vi "DDS_Clock.vi"() -> ()   [LabVIEW 2016] (continued)
{"STEP"=0, "time[ms]"=0.05, "time tolerance[us]"=0.01, "CH0"=TRUE, "rel. amplitude CH0"=1.0, "phase [°] CH0"=0.0, "f0 [Hz] CH0"=304600000.0, "f1 [Hz] CH0"=304400000.0, "CH1"=FALSE, "rel. amplitude CH1"=1.0, "phase [°] CH1"=0.0, "f0 [Hz] CH1"=310000000.0, "f1 [Hz] CH1"=310000000.0}, {"STEP"=0, "time[ms]"=0.05, "time tolerance[us]"=0.01, "CH0"=TRUE, "rel. amplitude CH0"=1.0, "phase [°] CH0"=0.0, "f0 [Hz] CH0"=304400000.0, "f1 [Hz] CH0"=304200000.0, "CH1"=FALSE, "rel. amplitude CH1"=1.0, "phase [°] CH1"=0.0, "f0 [Hz] CH1"=310000000.0, "f1 [Hz] CH1"=310000000.0}, {"STEP"=0, "time[ms]"=0.05, "time tolerance[us]"=0.01, "CH0"=TRUE, "rel. amplitude CH0"=1.0, "phase [°] CH0"=0.0, "f0 [Hz] CH0"=304200000.0, "f1 [Hz] CH0"=304000000.0, "CH1"=FALSE, "rel. amplitude CH1"=1.0, "phase [°] CH1"=0.0, "f0 [Hz] CH1"=310000000.0, "f1 [Hz] CH1"=310000000.0}, {"STEP"=0, "time[ms]"=0.05, "time tolerance[us]"=0.01, "CH0"=TRUE, "rel. amplitude CH0"=1.0, "phase [°] CH0"=0.0, "f0 [Hz] CH0"=304000000.0, "f1 [Hz] CH0"=303800000.0, "CH1"=FALSE, "rel. amplitude CH1"=1.0, "phase [°] CH1"=0.0, "f0 [Hz] CH1"=310000000.0, "f1 [Hz] CH1"=310000000.0}, {"STEP"=0, "time[ms]"=0.05, "time tolerance[us]"=0.01, "CH0"=TRUE, "rel. amplitude CH0"=1.0, "phase [°] CH0"=0.0, "f0 [Hz] CH0"=303800000.0, "f1 [Hz] CH0"=303600000.0, "CH1"=FALSE, "rel. amplitude CH1"=1.0, "phase [°] CH1"=0.0, "f0 [Hz] CH1"=310000000.0, "f1 [Hz] CH1"=310000000.0}, {"STEP"=0, "time[ms]"=0.05, "time tolerance[us]"=0.01, "CH0"=TRUE, "rel. amplitude CH0"=1.0, "phase [°] CH0"=0.0, "f0 [Hz] CH0"=303600000.0, "f1 [Hz] CH0"=303399999.99999994, "CH1"=FALSE, "rel. amplitude CH1"=1.0, "phase [°] CH1"=0.0, "f0 [Hz] CH1"=310000000.0, "f1 [Hz] CH1"=310000000.0}, {"STEP"=0, "time[ms]"=0.05, "time tolerance[us]"=0.01, "CH0"=TRUE, "rel. amplitude CH0"=1.0, "phase [°] CH0"=0.0, "f0 [Hz] CH0"=303399999.99999994, "f1 [Hz] CH0"=303200000.0, "CH1"=FALSE, "rel. amplitude CH1"=1.0, "phase [°] CH1"=0.0, "f0 [Hz] CH1"=310000000.0, "f1 [Hz] CH1"=310000000.0}, {"STEP"=0, "time[ms]"=0.05, "time tolerance[us]"=0.01, "CH0"=TRUE, "rel. amplitude CH0"=1.0, "phase [°] CH0"=0.0, "f0 [Hz] CH0"=303200000.0, "f1 [Hz] CH0"=303000000.0, "CH1"=FALSE, "rel. amplitude CH1"=1.0, "phase [°] CH1"=0.0, "f0 [Hz] CH1"=310000000.0, "f1 [Hz] CH1"=310000000.0}, {"STEP"=0, "time[ms]"=0.05, "time tolerance[us]"=0.01, "CH0"=TRUE, "rel. amplitude CH0"=1.0, "phase [°] CH0"=0.0, "f0 [Hz] CH0"=303000000.0, "f1 [Hz] CH0"=302800000.0, "CH1"=FALSE, "rel. amplitude CH1"=1.0, "phase [°] CH1"=0.0, "f0 [Hz] CH1"=310000000.0, "f1 [Hz] CH1"=310000000.0}, {"STEP"=0, "time[ms]"=0.05, "time tolerance[us]"=0.01, "CH0"=TRUE, "rel. amplitude CH0"=1.0, "phase [°] CH0"=0.0, "f0 [Hz] CH0"=302800000.0, "f1 [Hz] CH0"=302600000.0, "CH1"=FALSE, "rel. amplitude CH1"=1.0, "phase [°] CH1"=0.0, "f0 [Hz] CH1"=310000000.0, "f1 [Hz] CH1"=310000000.0}, {"STEP"=0, "time[ms]"=0.05, "time tolerance[us]"=0.01, "CH0"=TRUE, "rel. amplitude CH0"=1.0, "phase [°] CH0"=0.0, "f0 [Hz] CH0"=302600000.0, "f1 [Hz] CH0"=302399999.99999994, "CH1"=FALSE, "rel. amplitude CH1"=1.0, "phase [°] CH1"=0.0, "f0 [Hz] CH1"=310000000.0, "f1 [Hz] CH1"=310000000.0}, {"STEP"=0, "time[ms]"=0.05, "time tolerance[us]"=0.01, "CH0"=TRUE, "rel. amplitude CH0"=1.0, "phase [°] CH0"=0.0, "f0 [Hz] CH0"=302399999.99999994, "f1 [Hz] CH0"=302200000.0, "CH1"=FALSE, "rel. amplitude CH1"=1.0, "phase [°] CH1"=0.0, "f0 [Hz] CH1"=310000000.0, "f1 [Hz] CH1"=310000000.0}, {"STEP"=0, "time[ms]"=0.05, "time tolerance[us]"=0.01, "CH0"=TRUE, "rel. amplitude CH0"=1.0, "phase [°] CH0"=0.0, "f0 [Hz] CH0"=302200000.0, "f1 [Hz] CH0"=302000000.0, "CH1"=FALSE, "rel. amplitude CH1"=1.0, "phase [°] CH1"=0.0, "f0 [Hz] CH1"=310000000.0, "f1 [Hz] CH1"=310000000.0}, {"STEP"=0, "time[ms]"=0.05, "time tolerance[us]"=0.01, "CH0"=TRUE, "rel. amplitude CH0"=1.0, "phase [°] CH0"=0.0, "f0 [Hz] CH0"=302000000.0, "f1 [Hz] CH0"=301800000.0, "CH1"=FALSE, "rel. amplitude CH1"=1.0, "phase [°] CH1"=0.0, "f0 [Hz] CH1"=310000000.0, "f1 [Hz] CH1"=310000000.0}, {"STEP"=0, "time[ms]"=0.05, "time tolerance[us]"=0.01, "CH0"=TRUE, "rel. amplitude CH0"=1.0, "phase [°] CH0"=0.0, "f0 [Hz] CH0"=301800000.0, "f1 [Hz] CH0"=301600000.0, "CH1"=FALSE, "rel. amplitude CH1"=1.0, "phase [°] CH1"=0.0, "f0 [Hz] CH1"=310000000.0, "f1 [Hz] CH1"=310000000.0}, {"STEP"=0, "time[ms]"=0.05, "time tolerance[us]"=0.01, "CH0"=TRUE, "rel. amplitude CH0"=1.0, "phase [°] CH0"=0.0, "f0 [Hz] CH0"=301600000.0, "f1 [Hz] CH0"=301400000.0, "CH1"=FALSE, "rel. amplitude CH1"=1.0, "phase [°] CH1"=0.0, "f0 [Hz] CH1"=310000000.0, "f1 [Hz] CH1"=310000000.0}, {"STEP"=0, "time[ms]"=0.05, "time tolerance[us]"=0.01, "CH0"=TRUE, "rel. amplitude CH0"=1.0, "phase [°] CH0"=0.0, "f0 [Hz] CH0"=301400000.0, "f1 [Hz] CH0"=301200000.0, "CH1"=FALSE, "rel. amplitude CH1"=1.0, "phase [°] CH1"=0.0, "f0 [Hz] CH1"=310000000.0, "f1 [Hz] CH1"=310000000.0}, {"STEP"=0, "time[ms]"=0.05, "time tolerance[us]"=0.01, "CH0"=TRUE, "rel. amplitude CH0"=1.0, "phase [°] CH0"=0.0, "f0 [Hz] CH0"=301200000.0, "f1 [Hz] CH0"=301000000.0, "CH1"=FALSE, "rel. amplitude CH1"=1.0, "phase [°] CH1"=0.0, "f0 [Hz] CH1"=310000000.0, "f1 [Hz] CH1"=310000000.0}, {"STEP"=0, "time[ms]"=0.05, "time tolerance[us]"=0.01, "CH0"=TRUE, "rel. amplitude CH0"=1.0, "phase [°] CH0"=0.0, "f0 [Hz] CH0"=301000000.0, "f1 [Hz] CH0"=300800000.0, "CH1"=FALSE, "rel. amplitude CH1"=1.0, "phase [°] CH1"=0.0, "f0 [Hz] CH1"=310000000.0, "f1 [Hz] CH1"=310000000.0}, {"STEP"=0, "time[ms]"=0.05, "time tolerance[us]"=0.01, "CH0"=TRUE, "rel. amplitude CH0"=1.0, "phase [°] CH0"=0.0, "f0 [Hz] CH0"=300800000.0, "f1 [Hz] CH0"=300600000.0, "CH1"=FALSE, "rel. amplitude CH1"=1.0, "phase [°] CH1"=0.0, "f0 [Hz] CH1"=310000000.0, "f1 [Hz] CH1"=310000000.0}, {"STEP"=0, "time[ms]"=0.05, "time tolerance[us]"=0.01, "CH0"=TRUE, "rel. amplitude CH0"=1.0, "phase [°] CH0"=0.0, "f0 [Hz] CH0"=300600000.0, "f1 [Hz] CH0"=300400000.0, "CH1"=FALSE, "rel. amplitude CH1"=1.0, "phase [°] CH1"=0.0, "f0 [Hz] CH1"=310000000.0, "f1 [Hz] CH1"=310000000.0}, {"STEP"=0, "time[ms]"=0.05, "time tolerance[us]"=0.01, "CH0"=TRUE, "rel. amplitude CH0"=1.0, "phase [°] CH0"=0.0, "f0 [Hz] CH0"=300400000.0, "f1 [Hz] CH0"=300200000.0, "CH1"=FALSE, "rel. amplitude CH1"=1.0, "phase [°] CH1"=0.0, "f0 [Hz] CH1"=310000000.0, "f1 [Hz] CH1"=310000000.0}, {"STEP"=0, "time[ms]"=0.05, "time tolerance[us]"=0.01, "CH0"=TRUE, "rel. amplitude CH0"=1.0, "phase [°] CH0"=0.0, "f0 [Hz] CH0"=300200000.0, "f1 [Hz] CH0"=300000000.0, "CH1"=FALSE, "rel. amplitude CH1"=1.0, "phase [°] CH1"=0.0, "f0 [Hz] CH1"=310000000.0, "f1 [Hz] CH1"=310000000.0}, {"STEP"=0, "time[ms]"=0.05, "time tolerance[us]"=0.01, "CH0"=TRUE, "rel. amplitude CH0"=1.0, "phase [°] CH0"=0.0, "f0 [Hz] CH0"=300000000.0, "f1 [Hz] CH0"=300200000.00000006, "CH1"=FALSE, "rel. amplitude CH1"=1.0, "phase [°] CH1"=0.0, "f0 [Hz] CH1"=310000000.0, "f1 [Hz] CH1"=310000000.0}, {"STEP"=0, "time[ms]"=0.05, "time tolerance[us]"=0.01, "CH0"=TRUE, "rel. amplitude CH0"=1.0, "phase [°] CH0"=0.0, "f0 [Hz] CH0"=300200000.00000006, "f1 [Hz] CH0"=300400000.0, "CH1"=FALSE, "rel. amplitude CH1"=1.0, "phase [°] CH1"=0.0, "f0 [Hz] CH1"=310000000.0, "f1 [Hz] CH1"=310000000.0}, {"STEP"=0, "time[ms]"=0.05, "time tolerance[us]"=0.01, "CH0"=TRUE, "rel. amplitude CH0"=1.0, "phase [°] CH0"=0.0, "f0 [Hz] CH0"=300400000.0, "f1 [Hz] CH0"=300600000.0, "CH1"=FALSE, "rel. amplitude CH1"=1.0, "phase [°] CH1"=0.0, "f0 [Hz] CH1"=310000000.0, "f1 [Hz] CH1"=310000000.0}, {"STEP"=0, "time[ms]"=0.05, "time tolerance[us]"=0.01, "CH0"=TRUE, "rel. amplitude CH0"=1.0, "phase [°] CH0"=0.0, "f0 [Hz] CH0"=300600000.0, "f1 [Hz] CH0"=300800000.0, "CH1"=FALSE, "rel. amplitude CH1"=1.0, "phase [°] CH1"=0.0, "f0 [Hz] CH1"=310000000.0, "f1 [Hz] CH1"=310000000.0}, {"STEP"=0, "time[ms]"=0.05, "time tolerance[us]"=0.01, "CH0"=TRUE, "rel. amplitude CH0"=1.0, "phase [°] CH0"=0.0, "f0 [Hz] CH0"=300800000.0, "f1 [Hz] CH0"=301000000.0, "CH1"=FALSE, "rel. amplitude CH1"=1.0, "phase [°] CH1"=0.0, "f0 [Hz] CH1"=310000000.0, "f1 [Hz] CH1"=310000000.0}, {"STEP"=0, "time[ms]"=0.05, "time tolerance[us]"=0.01, "CH0"=TRUE, "rel. amplitude CH0"=1.0, "phase [°] CH0"=0.0, "f0 [Hz] CH0"=301000000.0, "f1 [Hz] CH0"=301200000.0, "CH1"=FALSE, "rel. amplitude CH1"=1.0, "phase [°] CH1"=0.0, "f0 [Hz] CH1"=310000000.0, "f1 [Hz] CH1"=310000000.0}, {"STEP"=0, "time[ms]"=0.05, "time tolerance[us]"=0.01, "CH0"=TRUE, "rel. amplitude CH0"=1.0, "phase [°] CH0"=0.0, "f0 [Hz] CH0"=301200000.0, "f1 [Hz] CH0"=301400000.0, "CH1"=FALSE, "rel. amplitude CH1"=1.0, "phase [°] CH1"=0.0, "f0 [Hz] CH1"=310000000.0, "f1 [Hz] CH1"=310000000.0}, {"STEP"=0, "time[ms]"=0.05, "time tolerance[us]"=0.01, "CH0"=TRUE, "rel. amplitude CH0"=1.0, "phase [°] CH0"=0.0, "f0 [Hz] CH0"=301400000.0, "f1 [Hz] CH0"=301600000.00000006, "CH1"=FALSE, "rel. amplitude CH1"=1.0, "phase [°] CH1"=0.0, "f0 [Hz] CH1"=310000000.0, "f1 [Hz] CH1"=310000000.0}, {"STEP"=0, "time[ms]"=0.05, "time tolerance[us]"=0.01, "CH0"=TRUE, "rel. amplitude CH0"=1.0, "phase [°] CH0"=0.0, "f0 [Hz] CH0"=301600000.00000006, "f1 [Hz] CH0"=301800000.00000006, "CH1"=FALSE, "rel. amplitude CH1"=1.0, "phase [°] CH1"=0.0, "f0 [Hz] CH1"=310000000.0, "f1 [Hz] CH1"=310000000.0}, {"STEP"=0, "time[ms]"=0.05, "time tolerance[us]"=0.01, "CH0"=TRUE, "rel. amplitude CH0"=1.0, "phase [°] CH0"=0.0, "f0 [Hz] CH0"=301800000.00000006, "f1 [Hz] CH0"=302000000.0, "CH1"=FALSE, "rel. amplitude CH1"=1.0, "phase [°] CH1"=0.0, "f0 [Hz] CH1"=310000000.0, "f1 [Hz] CH1"=310000000.0}, {"STEP"=0, "time[ms]"=0.05, "time tolerance[us]"=0.01, "CH0"=TRUE, "rel. amplitude CH0"=1.0, "phase [°] CH0"=0.0, "f0 [Hz] CH0"=302000000.0, "f1 [Hz] CH0"=302200000.0, "CH1"=FALSE, "rel. amplitude CH1"=1.0, "phase [°] CH1"=0.0, "f0 [Hz] CH1"=310000000.0, "f1 [Hz] CH1"=310000000.0}, {"STEP"=0, "time[ms]"=0.05, "time tolerance[us]"=0.01, "CH0"=TRUE, "rel. amplitude CH0"=1.0, "phase [°] CH0"=0.0, "f0 [Hz] CH0"=302200000.0, "f1 [Hz] CH0"=302400000.0, "CH1"=FALSE, "rel. amplitude CH1"=1.0, "phase [°] CH1"=0.0, "f0 [Hz] CH1"=310000000.0, "f1 [Hz] CH1"=310000000.0}, {"STEP"=0, "time[ms]"=0.05, "time tolerance[us]"=0.01, "CH0"=TRUE, "rel. amplitude CH0"=1.0, "phase [°] CH0"=0.0, "f0 [Hz] CH0"=302400000.0, "f1 [Hz] CH0"=302600000.0, "CH1"=FALSE, "rel. amplitude CH1"=1.0, "phase [°] CH1"=0.0, "f0 [Hz] CH1"=310000000.0, "f1 [Hz] CH1"=310000000.0}, {"STEP"=0, "time[ms]"=0.05, "time tolerance[us]"=0.01, "CH0"=TRUE, "rel. amplitude CH0"=1.0, "phase [°] CH0"=0.0, "f0 [Hz] CH0"=302600000.0, "f1 [Hz] CH0"=302800000.0, "CH1"=FALSE, "rel. amplitude CH1"=1.0, "phase [°] CH1"=0.0, "f0 [Hz] CH1"=310000000.0, "f1 [Hz] CH1"=310000000.0}, {"STEP"=0, "time[ms]"=0.05, "time tolerance[us]"=0.01, "CH0"=TRUE, "rel. amplitude CH0"=1.0, "phase [°] CH0"=0.0, "f0 [Hz] CH0"=302800000.0, "f1 [Hz] CH0"=303000000.0, "CH1"=FALSE, "rel. amplitude CH1"=1.0, "phase [°] CH1"=0.0, "f0 [Hz] CH1"=310000000.0, "f1 [Hz] CH1"=310000000.0}, {"STEP"=0, "time[ms]"=0.05, "time tolerance[us]"=0.01, "CH0"=TRUE, "rel. amplitude CH0"=1.0, "phase [°] CH0"=0.0, "f0 [Hz] CH0"=303000000.0, "f1 [Hz] CH0"=303200000.00000006, "CH1"=FALSE, "rel. amplitude CH1"=1.0, "phase [°] CH1"=0.0, "f0 [Hz] CH1"=310000000.0, "f1 [Hz] CH1"=310000000.0}, {"STEP"=0, "time[ms]"=0.05, "time tolerance[us]"=0.01, "CH0"=TRUE, "rel. amplitude CH0"=1.0, "phase [°] CH0"=0.0, "f0 [Hz] CH0"=303200000.00000006, "f1 [Hz] CH0"=303400000.0, "CH1"=FALSE, "rel. amplitude CH1"=1.0, "phase [°] CH1"=0.0, "f0 [Hz] CH1"=310000000.0, "f1 [Hz] CH1"=310000000.0}, {"STEP"=0, "time[ms]"=0.05, "time tolerance[us]"=0.01, "CH0"=TRUE, "rel. amplitude CH0"=1.0, "phase [°] CH0"=0.0, "f0 [Hz] CH0"=303400000.0, "f1 [Hz] CH0"=303600000.0, "CH1"=FALSE, "rel. amplitude CH1"=1.0, "phase [°] CH1"=0.0, "f0 [Hz] CH1"=310000000.0, "f1 [Hz] CH1"=310000000.0}, {"STEP"=0, "time[ms]"=0.05, "time tolerance[us]"=0.01, "CH0"=TRUE, "rel. amplitude CH0"=1.0, "phase [°] CH0"=0.0, "f0 [Hz] CH0"=303600000.0, "f1 [Hz] CH0"=303800000.0, "CH1"=FALSE, "rel. amplitude CH1"=1.0, "phase [°] CH1"=0.0, "f0 [Hz] CH1"=310000000.0, "f1 [Hz] CH1"=310000000.0}, {"STEP"=0, "time[ms]"=0.05, "time tolerance[us]"=0.01, "CH0"=TRUE, "rel. amplitude CH0"=1.0, "phase [°] CH0"=0.0, "f0 [Hz] CH0"=303800000.0, "f1 [Hz] CH0"=304000000.0, "CH1"=FALSE, "rel. amplitude CH1"=1.0, "phase [°] CH1"=0.0, "f0 [Hz] CH1"=310000000.0, "f1 [Hz] CH1"=310000000.0}, {"STEP"=0, "time[ms]"=0.05, "time tolerance[us]"=0.01, "CH0"=TRUE, "rel. amplitude CH0"=1.0, "phase [°] CH0"=0.0, "f0 [Hz] CH0"=304000000.0, "f1 [Hz] CH0"=304200000.0, "CH1"=FALSE, "rel. amplitude CH1"=1.0, "phase [°] CH1"=0.0, "f0 [Hz] CH1"=310000000.0, "f1 [Hz] CH1"=310000000.0}, {"STEP"=0, "time[ms]"=0.05, "time tolerance[us]"=0.01, "CH0"=TRUE, "rel. amplitude CH0"=1.0, "phase [°] CH0"=0.0, "f0 [Hz] CH0"=304200000.0, "f1 [Hz] CH0"=304400000.0, "CH1"=FALSE, "rel. amplitude CH1"=1.0, "phase [°] CH1"=0.0, "f0 [Hz] CH1"=310000000.0, "f1 [Hz] CH1"=310000000.0}, {"STEP"=0, "time[ms]"=0.05, "time tolerance[us]"=0.01, "CH0"=TRUE, "rel. amplitude CH0"=1.0, "phase [°] CH0"=0.0, "f0 [Hz] CH0"=304400000.0, "f1 [Hz] CH0"=304600000.00000006, "CH1"=FALSE, "rel. amplitude CH1"=1.0, "phase [°] CH1"=0.0, "f0 [Hz] CH1"=310000000.0, "f1 [Hz] CH1"=310000000.0}, {"STEP"=0, "time[ms]"=0.05, "time tolerance[us]"=0.01, "CH0"=TRUE, "rel. amplitude CH0"=1.0, "phase [°] CH0"=0.0, "f0 [Hz] CH0"=304600000.00000006, "f1 [Hz] CH0"=304800000.0, "CH1"=FALSE, "rel. amplitude CH1"=1.0, "phase [°] CH1"=0.0, "f0 [Hz] CH1"=310000000.0, "f1 [Hz] CH1"=310000000.0}, {"STEP"=0, "time[ms]"=0.05, "time tolerance[us]"=0.01, "CH0"=TRUE, "rel. amplitude CH0"=1.0, "phase [°] CH0"=0.0, "f0 [Hz] CH0"=304800000.0, "f1 [Hz] CH0"=305000000.0, "CH1"=FALSE, "rel. amplitude CH1"=1.0, "phase [°] CH1"=0.0, "f0 [Hz] CH1"=310000000.0, "f1 [Hz] CH1"=310000000.0}, {"STEP"=0, "time[ms]"=0.05, "time tolerance[us]"=0.01, "CH0"=TRUE, "rel. amplitude CH0"=1.0, "phase [°] CH0"=0.0, "f0 [Hz] CH0"=305000000.0, "f1 [Hz] CH0"=305200000.00000006, "CH1"=FALSE, "rel. amplitude CH1"=1.0, "phase [°] CH1"=0.0, "f0 [Hz] CH1"=310000000.0, "f1 [Hz] CH1"=310000000.0}, {"STEP"=0, "time[ms]"=0.05, "time tolerance[us]"=0.01, "CH0"=TRUE, "rel. amplitude CH0"=1.0, "phase [°] CH0"=0.0, "f0 [Hz] CH0"=305200000.00000006, "f1 [Hz] CH0"=305400000.0, "CH1"=FALSE, "rel. amplitude CH1"=1.0, "phase [°] CH1"=0.0, "f0 [Hz] CH1"=310000000.0, "f1 [Hz] CH1"=310000000.0}, {"STEP"=0, "time[ms]"=0.05, "time tolerance[us]"=0.01, "CH0"=TRUE, "rel. amplitude CH0"=1.0, "phase [°] CH0"=0.0, "f0 [Hz] CH0"=305400000.0, "f1 [Hz] CH0"=305600000.0, "CH1"=FALSE, "rel. amplitude CH1"=1.0, "phase [°] CH1"=0.0, "f0 [Hz] CH1"=310000000.0, "f1 [Hz] CH1"=310000000.0}, {"STEP"=0, "time[ms]"=0.05, "time tolerance[us]"=0.01, "CH0"=TRUE, "rel. amplitude CH0"=1.0, "phase [°] CH0"=0.0, "f0 [Hz] CH0"=305600000.0, "f1 [Hz] CH0"=305800000.0, "CH1"=FALSE, "rel. amplitude CH1"=1.0, "phase [°] CH1"=0.0, "f0 [Hz] CH1"=310000000.0, "f1 [Hz] CH1"=310000000.0}, {"STEP"=0, "time[ms]"=0.05, "time tolerance[us]"=0.01, "CH0"=TRUE, "rel. amplitude CH0"=1.0, "phase [°] CH0"=0.0, "f0 [Hz] CH0"=305800000.0, "f1 [Hz] CH0"=306000000.0, "CH1"=FALSE, "rel. amplitude CH1"=1.0, "phase [°] CH1"=0.0, "f0 [Hz] CH1"=310000000.0, "f1 [Hz] CH1"=310000000.0}, {"STEP"=0, "time[ms]"=0.05, "time tolerance[us]"=0.01, "CH0"=TRUE, "rel. amplitude CH0"=1.0, "phase [°] CH0"=0.0, "f0 [Hz] CH0"=306000000.0, "f1 [Hz] CH0"=306200000.0, "CH1"=FALSE, "rel. amplitude CH1"=1.0, "phase [°] CH1"=0.0, "f0 [Hz] CH1"=310000000.0, "f1 [Hz] CH1"=310000000.0}, {"STEP"=0, "time[ms]"=0.05, "time tolerance[us]"=0.01, "CH0"=TRUE, "rel. amplitude CH0"=1.0, "phase [°] CH0"=0.0, "f0 [Hz] CH0"=306200000.0, "f1 [Hz] CH0"=306400000.0, "CH1"=FALSE, "rel. amplitude CH1"=1.0, "phase [°] CH1"=0.0, "f0 [Hz] CH1"=310000000.0, "f1 [Hz] CH1"=310000000.0}, {"STEP"=0, "time[ms]"=0.05, "time tolerance[us]"=0.01, "CH0"=TRUE, "rel. amplitude CH0"=1.0, "phase [°] CH0"=0.0, "f0 [Hz] CH0"=306400000.0, "f1 [Hz] CH0"=306600000.00000006, "CH1"=FALSE, "rel. amplitude CH1"=1.0, "phase [°] CH1"=0.0, "f0 [Hz] CH1"=310000000.0, "f1 [Hz] CH1"=310000000.0}, {"STEP"=0, "time[ms]"=0.05, "time tolerance[us]"=0.01, "CH0"=TRUE, "rel. amplitude CH0"=1.0, "phase [°] CH0"=0.0, "f0 [Hz] CH0"=306600000.00000006, "f1 [Hz] CH0"=306800000.00000006, "CH1"=FALSE, "rel. amplitude CH1"=1.0, "phase [°] CH1"=0.0, "f0 [Hz] CH1"=310000000.0, "f1 [Hz] CH1"=310000000.0}, {"STEP"=0, "time[ms]"=0.05, "time tolerance[us]"=0.01, "CH0"=TRUE, "rel. amplitude CH0"=1.0, "phase [°] CH0"=0.0, "f0 [Hz] CH0"=306800000.00000006, "f1 [Hz] CH0"=307000000.0, "CH1"=FALSE, "rel. amplitude CH1"=1.0, "phase [°] CH1"=0.0, "f0 [Hz] CH1"=310000000.0, "f1 [Hz] CH1"=310000000.0}, {"STEP"=0, "time[ms]"=0.05, "time tolerance[us]"=0.01, "CH0"=TRUE, "rel. amplitude CH0"=1.0, "phase [°] CH0"=0.0, "f0 [Hz] CH0"=307000000.0, "f1 [Hz] CH0"=307200000.0, "CH1"=FALSE, "rel. amplitude CH1"=1.0, "phase [°] CH1"=0.0, "f0 [Hz] CH1"=310000000.0, "f1 [Hz] CH1"=310000000.0}, {"STEP"=0, "time[ms]"=0.05, "time tolerance[us]"=0.01, "CH0"=TRUE, "rel. amplitude CH0"=1.0, "phase [°] CH0"=0.0, "f0 [Hz] CH0"=307200000.0, "f1 [Hz] CH0"=307400000.0, "CH1"=FALSE, "rel. amplitude CH1"=1.0, "phase [°] CH1"=0.0, "f0 [Hz] CH1"=310000000.0, "f1 [Hz] CH1"=310000000.0}, {"STEP"=0, "time[ms]"=0.05, "time tolerance[us]"=0.01, "CH0"=TRUE, "rel. amplitude CH0"=1.0, "phase [°] CH0"=0.0, "f0 [Hz] CH0"=307400000.0, "f1 [Hz] CH0"=307600000.0, "CH1"=FALSE, "rel. amplitude CH1"=1.0, "phase [°] CH1"=0.0, "f0 [Hz] CH1"=310000000.0, "f1 [Hz] CH1"=310000000.0}, {"STEP"=0, "time[ms]"=0.05, "time tolerance[us]"=0.01, "CH0"=TRUE, "rel. amplitude CH0"=1.0, "phase [°] CH0"=0.0, "f0 [Hz] CH0"=307600000.0, "f1 [Hz] CH0"=307800000.0, "CH1"=FALSE, "rel. amplitude CH1"=1.0, "phase [°] CH1"=0.0, "f0 [Hz] CH1"=310000000.0, "f1 [Hz] CH1"=310000000.0}, {"STEP"=0, "time[ms]"=0.05, "time tolerance[us]"=0.01, "CH0"=TRUE, "rel. amplitude CH0"=1.0, "phase [°] CH0"=0.0, "f0 [Hz] CH0"=307800000.0, "f1 [Hz] CH0"=308000000.0, "CH1"=FALSE, "rel. amplitude CH1"=1.0, "phase [°] CH1"=0.0, "f0 [Hz] CH1"=310000000.0, "f1 [Hz] CH1"=310000000.0}, {"STEP"=0, "time[ms]"=0.05, "time tolerance[us]"=0.01, "CH0"=TRUE, "rel. amplitude CH0"=1.0, "phase [°] CH0"=0.0, "f0 [Hz] CH0"=308000000.0, "f1 [Hz] CH0"=308200000.00000006, "CH1"=FALSE, "rel. amplitude CH1"=1.0, "phase [°] CH1"=0.0, "f0 [Hz] CH1"=310000000.0, "f1 [Hz] CH1"=310000000.0}, {"STEP"=0, "time[ms]"=0.05, "time tolerance[us]"=0.01, "CH0"=TRUE, "rel. amplitude CH0"=1.0, "phase [°] CH0"=0.0, "f0 [Hz] CH0"=308200000.00000006, "f1 [Hz] CH0"=308400000.0, "CH1"=FALSE, "rel. amplitude CH1"=1.0, "phase [°] CH1"=0.0, "f0 [Hz] CH1"=310000000.0, "f1 [Hz] CH1"=310000000.0}, {"STEP"=0, "time[ms]"=0.05, "time tolerance[us]"=0.01, "CH0"=TRUE, "rel. amplitude CH0"=1.0, "phase [°] CH0"=0.0, "f0 [Hz] CH0"=308400000.0, "f1 [Hz] CH0"=308600000.0, "CH1"=FALSE, "rel. amplitude CH1"=1.0, "phase [°] CH1"=0.0, "f0 [Hz] CH1"=310000000.0, "f1 [Hz] CH1"=310000000.0}, {"STEP"=0, "time[ms]"=0.05, "time tolerance[us]"=0.01, "CH0"=TRUE, "rel. amplitude CH0"=1.0, "phase [°] CH0"=0.0, "f0 [Hz] CH0"=308600000.0, "f1 [Hz] CH0"=308800000.0, "CH1"=FALSE, "rel. amplitude CH1"=1.0, "phase [°] CH1"=0.0, "f0 [Hz] CH1"=310000000.0, "f1 [Hz] CH1"=310000000.0}, {"STEP"=0, "time[ms]"=0.05, "time tolerance[us]"=0.01, "CH0"=TRUE, "rel. amplitude CH0"=1.0, "phase [°] CH0"=0.0, "f0 [Hz] CH0"=308800000.0, "f1 [Hz] CH0"=309000000.0, "CH1"=FALSE, "rel. amplitude CH1"=1.0, "phase [°] CH1"=0.0, "f0 [Hz] CH1"=310000000.0, "f1 [Hz] CH1"=310000000.0}, {"STEP"=0, "time[ms]"=0.05, "time tolerance[us]"=0.01, "CH0"=TRUE, "rel. amplitude CH0"=1.0, "phase [°] CH0"=0.0, "f0 [Hz] CH0"=309000000.0, "f1 [Hz] CH0"=309200000.0, "CH1"=FALSE, "rel. amplitude CH1"=1.0, "phase [°] CH1"=0.0, "f0 [Hz] CH1"=310000000.0, "f1 [Hz] CH1"=310000000.0}, {"STEP"=0, "time[ms]"=0.05, "time tolerance[us]"=0.01, "CH0"=TRUE, "rel. amplitude CH0"=1.0, "phase [°] CH0"=0.0, "f0 [Hz] CH0"=309200000.0, "f1 [Hz] CH0"=309400000.0, "CH1"=FALSE, "rel. amplitude CH1"=1.0, "phase [°] CH1"=0.0, "f0 [Hz] CH1"=310000000.0, "f1 [Hz] CH1"=310000000.0}, {"STEP"=0, "time[ms]"=0.05, 
